vi "JSR SetAll.vi"(8 "error in (no error)":errorcluster, 10 "JSR Complete":T1={"JSR Pulse Settings"={"Damping"=59, "Pulse Energy Level"=2, "Pulser Impedance"=0, "Pulser Voltage (V)"=100}, "JSR Receive Settings"={"Receiver Mode"=0, "High Pass Filter"=5000, "Low Pass Filter"=50, "Gain (dB)"=50}, "JSR Trigger Settings"={"External Trigger Limit"=0, "Trigger Source"=1, "PRF (Hz)"=1.75}} {"JSR Trigger Settings"."PRF (Hz)" items=["100 Hz"=0.1, "200 Hz"=0.2, "400 Hz"=0.4, "600 Hz"=0.6, "800 Hz"=0.8, "1000 Hz"=1.0, "1250 Hz"=1.25, "1500 Hz"=1.5, "1750 Hz"=1.75, "2000 Hz"=2.0, "2500 Hz"=2.5, "3000 Hz"=3.0, "3500 Hz"=3.5, "4000 Hz"=4.0, "4500 Hz"=4.5, "5000 Hz"=5.0]; "JSR Trigger Settings"."Trigger Source" items=["Internal", "External"]; "JSR Trigger Settings"."External Trigger Limit" items=["No Limit", "5 kHz"]; "JSR Receive Settings"."Gain (dB)" min=-13 max=66 step=1; "JSR Receive Settings"."Low Pass Filter" items=["5 MHz"=5, "10 MHz"=10, "15 MHz"=15, "22.5 MHz"=22, "35 MHz"=35, "50 MHz"=50]; "JSR Receive Settings"."High Pass Filter" items=["DC"=0, "1 MHz"=1000, "2.5 MHz"=2500, "5 MHz"=5000, "7.5 MHz"=7500, "12.5 MHz"=12500]; "JSR Receive Settings"."Receiver Mode" items=["Echo", "Through"]; "JSR Pulse Settings"."Pulser Voltage (V)" items=["100"=100, "125"=125, "150"=150, "175"=175, "200"=200, "225"=225, "250"=250, "275"=275, "300"=300, "325"=325, "350"=350, "375"=375, "400"=400, "425"=425, "450"=450, "475"=475]; "JSR Pulse Settings"."Pulser Impedance" items=["High z", "Low z"]; "JSR Pulse Settings"."Pulse Energy Level" items=["0 (Minimum)", "1", "2", "3 (Maximum)"]; "JSR Pulse Settings"."Damping" items=["331 Ohms"=331, "198 Ohms"=198, "142 Ohms"=142, "110 Ohms"=110, "92 Ohms"=92, "77 Ohms"=77, "67 Ohms"=67, "59 Ohms"=59, "52 Ohms"=52, "47 Ohms"=47, "43 Ohms"=43, "39 Ohms"=39, "37 Ohms"=37, "34 Ohms"=34, "32 Ohms"=32, "30 Ohms"=30]}, 11 "JSR VISA":refnum<visa-resource-name>) -> (0 "error out":errorcluster, 3 "JSR VISA Out":refnum<visa-resource-name>)   [LabVIEW 2022 SP3]
uses:
  Controls/JSR Complete.ctl
  Controls/JSR Pulse.ctl
  Controls/Damping.ctl
  Controls/Energy.ctl
  Controls/Z.ctl
  Controls/Volt.ctl
  Controls/JSR Recieve.ctl
  Controls/Mode.ctl
  Controls/HPF.ctl
  Controls/LPF.ctl
  Controls/Gain.ctl
  Controls/JSR Trigger.ctl
  Controls/Trig Limit.ctl
  Controls/Trig Source.ctl
  Controls/PRF.ctl
  PulserGlobals.vi
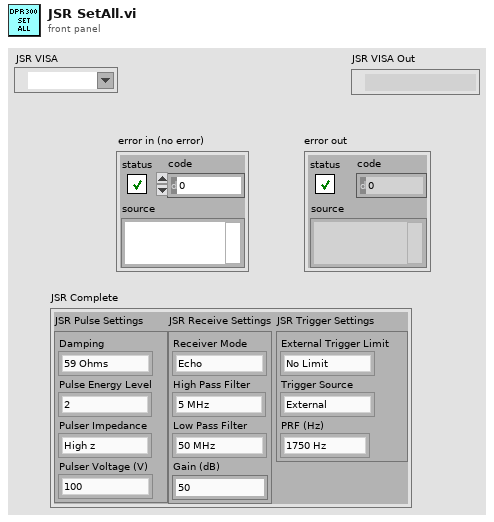
[diagram p1: front panel]
types:
  T1 = typedef "JSR Complete.ctl" = cluster{"JSR Pulse Settings":T2, "JSR Receive Settings":T7, "JSR Trigger Settings":T12}
  T2 = typedef "JSR Pulse.ctl" = cluster{"Damping":T3, "Pulse Energy Level":T4, "Pulser Impedance":T5, "Pulser Voltage (V)":T6}
  T3 = typedef "Damping.ctl" = i16
  T4 = typedef "Energy.ctl" = u16
  T5 = typedef "Z.ctl" = u16
  T6 = typedef "Volt.ctl" = i16
  T7 = typedef "JSR Recieve.ctl" = cluster{"Receiver Mode":T8, "High Pass Filter":T9, "Low Pass Filter":T10, "Gain (dB)":T11}
  T8 = typedef "Mode.ctl" = i8
  T9 = typedef "HPF.ctl" = u16
  T10 = typedef "LPF.ctl" = u16
  T11 = typedef "Gain.ctl" = i8
  T12 = typedef "JSR Trigger.ctl" = cluster{"External Trigger Limit":T13, "Trigger Source":T14, "PRF (Hz)":T15}
  T13 = typedef "Trig Limit.ctl" = i8
  T14 = typedef "Trig Source.ctl" = i8
  T15 = typedef "PRF.ctl" = dbl
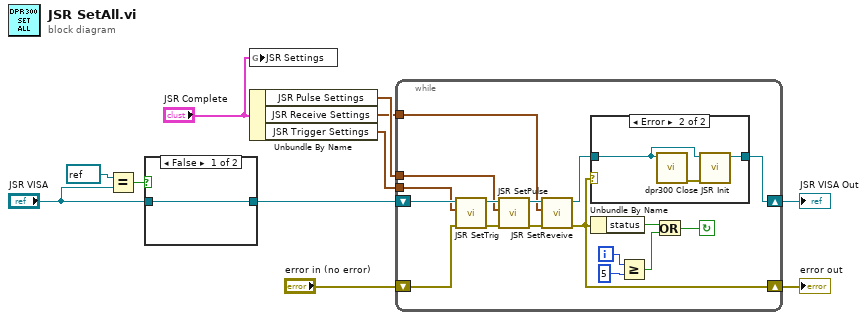
[diagram p0: block diagram]
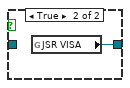
[diagram p3: hidden frame]
diagram:
  n1 = Equal?(x=refnum<visa-resource-name> refnum, y="JSR VISA") -> (x = y?=w5:bool)
  n2 = case shown="False" w5 {
    tunnel: [w12 w13] -> w8
    tunnel: "JSR VISA" -> [w12 _]
    frame False {
    }
    frame True {
      n3 = global read "PulserGlobals.vi" "JSR VISA"() -> (w13:refnum<visa-resource-name>)
    }
  }
  n4 = global write "PulserGlobals.vi" "JSR Settings"("JSR Complete") -> ()
  n5 = Unbundle By Name("JSR Complete") -> ("JSR Pulse Settings"=w4:T2, "JSR Receive Settings"=w3:T7, "JSR Trigger Settings"=w2:T12)
  n6 = while {
    tunnel: w4 -> [w24]
    tunnel: w3 -> [w23]
    tunnel: w2 -> [w22]
    shift-right: [w21] -> w9
    shift-left: "error in (no error)" -> [w30]
    shift-right: [w19] -> w10
    shift-left: w8 -> [w25]
    i -> [w18]
    stop <- w16 continue-if-true
    n7 = call "JSR SetTrig.vi"("error in (no error)"=w30, "JSR Trigger Settings"=w22, "VISA Refnum in"=w25) -> ("error out"=w26:errorcluster, "VISA Refnum out"=w27:refnum<visa-resource-name>)  [unwired: 7 in]
    n8 = call "JSR SetPulse.vi"("error in (no error)"=w26, "JSR Pulse Settings"=w24, "VISA Refnum in"=w27) -> ("error out"=w29:errorcluster, "VISA Refnum out"=w28:refnum<visa-resource-name>)  [unwired: 7 in]
    n9 = call "JSR SetReveive.vi"("error in (no error)"=w29, "JSR Receive Settings"=w23, "VISA Refnum in"=w28) -> ("error out"=w21:errorcluster, "VISA Refnum out"=w20:refnum<visa-resource-name>)  [unwired: 7 in]
    n10 = case shown="Error" w21 {
      tunnel: w20 -> [w31 w32]
      tunnel: [w31 w33] -> w19
      frame No Error {
      }
      frame Error {
        n11 = call <instrlib>:"dpr300 Close.vi"("VISA resource name"=w32) -> ("error out"=w34:errorcluster)  [unwired: 10 in]
        n12 = call "JSR Init.vi"("error in (no error)"=w34, "JSR VISA"=w32) -> ("JSR VISA Out"=w33:refnum<visa-resource-name>)  [unwired: 8 in, 1 out]
      }
    }
    n13 = Unbundle By Name(w21) -> ("status"=w14:bool)
    n14 = Greater Or Equal?(x=w18, y=5) -> (x >= y?=w15:bool)
    n15 = Or(x=w14, y=w15) -> (x .or. y?=w16:bool)
  }
  "error out" <- w9
  "JSR VISA Out" <- w10
